vi "Output Timing.vi"(4 "Min On":dbl, 6 "Cycle":dbl, 7 "HRS Time":dbl, 8 "error in (no error)":errorcluster, 10 "Out 0-1":dbl, 11 "TimedPWMControl in":refnum<class "TimedPWMControl.lvclass">) -> (0 "error out":errorcluster, 2 "Output":bool, 3 "TimedPWMControl out":refnum<class "TimedPWMControl.lvclass">)   [LabVIEW 2020, in "VolatusControl.lvlib" / "TimedPWMControl.lvclass"]
uses:
  TimedPWMControl.lvclass
  TimedPWMControl.lvclass/TimedPWMControl.ctl
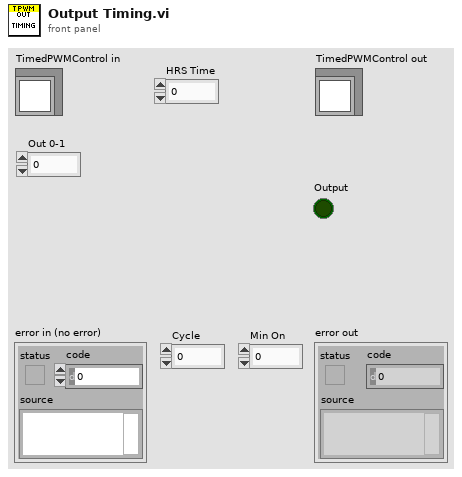
[diagram p1: front panel]
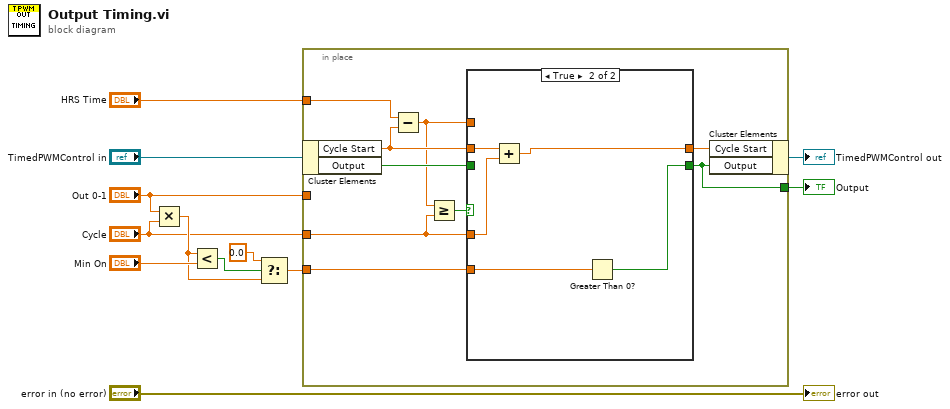
[diagram p0: block diagram]
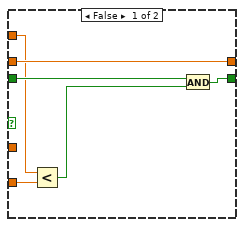
[diagram p2: hidden frame]
diagram:
  n1 = Multiply(x="Out 0-1", y="Cycle") -> (x*y=w10:dbl)
  n2 = Less?(x=w10, y="Min On") -> (x < y?=w9:bool)
  n3 = Select(t=0.0, s=w9, f=w10) -> (s? t:f=w6:dbl)
  n4 = in-place {
    in-place-border: w6 -> [w20]
    in-place-border: "Cycle" -> [w13]
    in-place-border: "Out 0-1" -> [_]
    in-place-border: "HRS Time" -> [w21]
    in-place-border: [w15] -> w2
    n5 = in-place-cluster #1("TimedPWMControl in") -> ("Cycle Start"=w17:dbl, "Output"=w18:bool)
    n6 = Subtract(x=w21, y=w17) -> (x-y=w14:dbl)
    n7 = Greater Or Equal?(x=w14, y=w13) -> (x >= y?=w19:bool)
    n8 = case shown="True" w19 {
      tunnel: w20 -> [w24 w32]
      tunnel: w18 -> [w26 _]
      tunnel: w17 -> [w27 w30]
      tunnel: [w27 w28] -> w16
      tunnel: [w25 w31] -> w15
      tunnel: w14 -> [w23 _]
      tunnel: w13 -> [_ w29]
      frame False {
        n9 = Less?(x=w23, y=w24) -> (x < y?=w22:bool)
        n10 = And(x=w26, y=w22) -> (x .and. y?=w25:bool)
      }
      frame True {
        n11 = Add(x=w30, y=w29) -> (x+y=w28:dbl)
        n12 = Greater Than 0?(x=w32) -> (x > 0?=w31:bool)
      }
    }
    n13 = in-place-cluster #1("Cycle Start"=w16, "Output"=w15) -> (→"TimedPWMControl out":refnum<class "TimedPWMControl.lvclass">)
  }
  "Output" <- w2
  "error out" <- "error in (no error)"
